vi "AR-Interlock-monitor.vi"() -> ()   [LabVIEW 2021]
uses:
  <vilib>/Instr/_visa.llb/VISA Flush IO Buffer Mask.ctl
panel:
  out "Output":string
  in  "Read":bool
  in  "stop":bool
  in  "Inlk Com":refnum<visa-resource-name>
  in  "error in":errorcluster
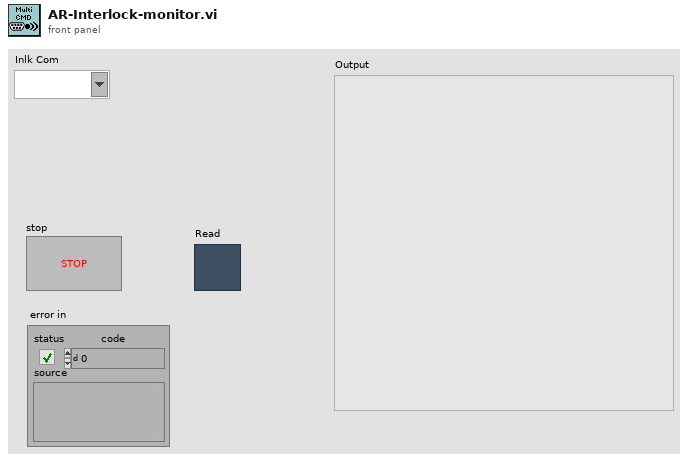
[diagram p1: front panel]
types:
  T1 = cluster{"Baud Rate":u32, "Parity":u16, "Data Bits":u16, "Serial Settings:Serial Flow Control":u16, "Serial Port":u16, "Serial Settings:Serial Stop Bits":u16}
  T2 = typedef "VISA Flush IO Buffer Mask.ctl" = u16
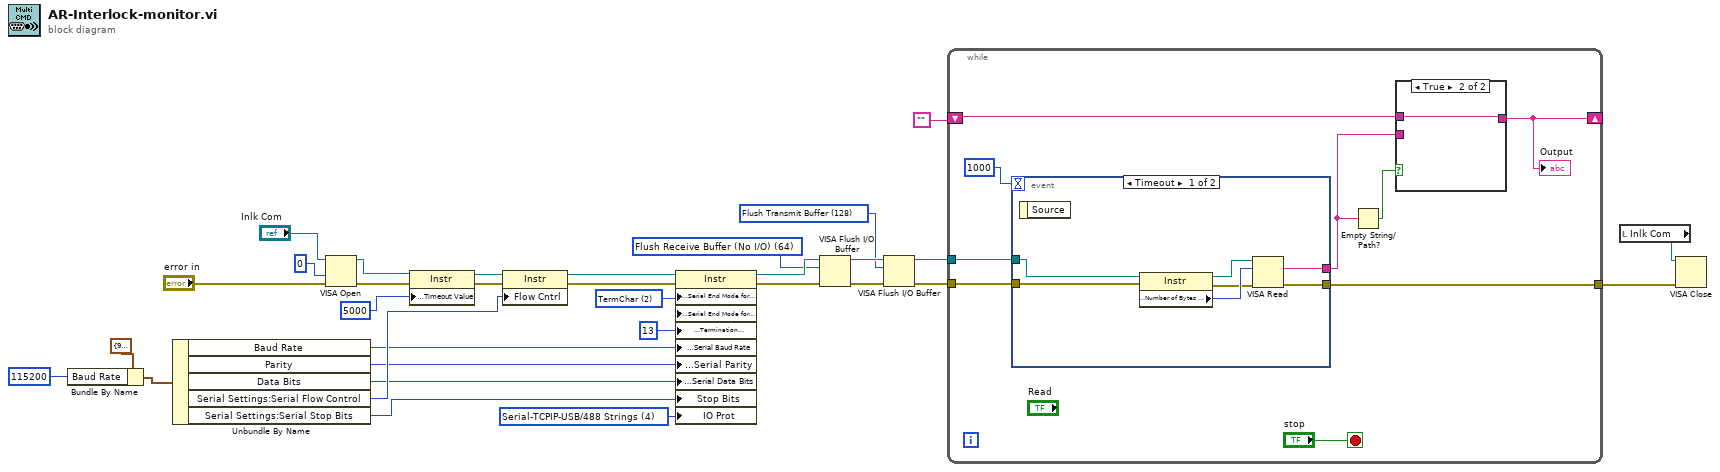
[diagram p0: block diagram]
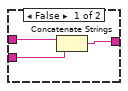
[diagram p2: hidden frame]
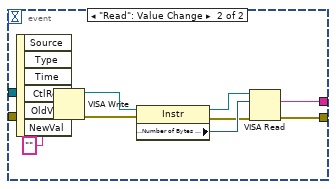
[diagram p3: hidden frame]
diagram:
  w7 = T2 128 items=["Flush Receive Buffer"=16, "Write Transmit Buffer to Device"=32, "Flush Receive Buffer (No I/O)"=64, "Flush Transmit Buffer"=128] ("Mask")
  w12 = T2 64 items=["Flush Receive Buffer"=16, "Write Transmit Buffer to Device"=32, "Flush Receive Buffer (No I/O)"=64, "Flush Transmit Buffer"=128] ("Mask")
  w23 = u16 2 items=["None", "LastBit", "TermChar"] ("Serial Settings:Serial End Mode for Reads")
  w19 = u16 4 items=["Normal"=1, "VXI/FDC"=2, "GPIB/HS488"=3, "Serial-TCPIP-USB/488 Strings"=4, "USBTMC/Vendor-Specific"=5] ("Message Based Settings:IO Protocol")
  n1 = Bundle By Name(cluster=T1 {"Baud Rate"=9600, "Parity"=0, "Data Bits"=8, "Serial Settings:Serial Flow Control"=0, "Serial Port"=6, "Serial Settings:Serial Stop Bits"=10} ("Serial Configuration"), "Baud Rate"=u32 115200) -> (w15:T1)
  n2 = Unbundle By Name(w15) -> ("Baud Rate"=w22:u32, "Parity"=w21:u16, "Data Bits"=w20:u16, "Serial Settings:Serial Flow Control"=w26:u16, "Serial Settings:Serial Stop Bits"=w18:u16)
  n3 = VISA Open(access mode=u32 0, error in (no error)="error in", VISA resource name="Inlk Com") -> (VISA resource name=w30:refnum<visa-resource-name>, error out=w31:errorcluster)  [unwired: 2 in]
  n4 = property on="Property Node" class="Instr"(reference=w30, error in=w31, "General Settings:Timeout Value"=u32 5000 ("Timeout [ms]")) -> (reference out=w28:refnum<visa-resource-name>, error out=w27:errorcluster)
  n5 = property on="Property Node" class="Instr"(reference=w28, error in=w27, "Flow Cntrl"=w26) -> (reference out=w25:refnum<visa-resource-name>, error out=w24:errorcluster)
  n6 = property on="Property Node" class="Instr"(reference=w25, error in=w24, "Serial Settings:Serial End Mode for Reads"=w23, "Serial Settings:Serial End Mode for Writes"=w23, "Message Based Settings:Termination Character"=u8 13, "Serial Settings:Serial Baud Rate"=w22, "Serial Settings:Serial Parity"=w21, "Serial Settings:Serial Data Bits"=w20, "Stop Bits"=w18, "IO Prot"=w19) -> (reference out=w14:refnum<visa-resource-name>, error out=w13:errorcluster)
  n7 = VISA Flush I/O Buffer(VISA resource name=w14, mask (16)=w12, error in (no error)=w13) -> (VISA resource name out=w11:refnum<visa-resource-name>, error out=w10:errorcluster)
  n8 = VISA Flush I/O Buffer(VISA resource name=w11, mask (16)=w7, error in (no error)=w10) -> (VISA resource name out=w8:refnum<visa-resource-name>, error out=w9:errorcluster)
  n9 = while {
    tunnel: w9 -> [w41]
    tunnel: w8 -> [w40]
    tunnel: [w37] -> w2
    shift-right: [w33] -> _
    shift-left: "" -> [w34]
    stop <- "stop" stop-if-true
    n10 = event shown="[0] Timeout" {
      selector: _ -> [_ _]
      dyn-events: _ -> [_ _]
      timeout: 1000 -> [_ _]
      tunnel: w41 -> [w49 w62]
      tunnel: w40 -> [w48 w61]
      tunnel: [w47 w55] -> w37
      tunnel: [w46 w54] -> w35
      event Timeout {
        n11 = event-data() -> ()  [unwired: 1 in, 1 out]
        n12 = property class="Instr"(reference=w48, error in=w49) -> (reference out=w52:refnum<visa-resource-name>, error out=w50:errorcluster, "Serial Settings:Number of Bytes at Serial Port"=w51:u32)
        n13 = VISA Read(VISA resource name=w52, byte count=w51, error in (no error)=w50) -> (read buffer=w46:string, error out=w47:errorcluster)  [unwired: 2 out]
      }
      event "Read": Value Change {
        n14 = event-data() -> ()  [unwired: 1 in, 6 out]
        n15 = VISA Write(VISA resource name=w61, write buffer="", error in (no error)=w62) -> (VISA resource name out=w60:refnum<visa-resource-name>, error out=w59:errorcluster)  [unwired: 1 out]
        n16 = property class="Instr"(reference=w60, error in=w59) -> (reference out=w58:refnum<visa-resource-name>, error out=w56:errorcluster, "Serial Settings:Number of Bytes at Serial Port"=w57:u32)
        n17 = VISA Read(VISA resource name=w58, byte count=w57, error in (no error)=w56) -> (read buffer=w54:string, error out=w55:errorcluster)  [unwired: 2 out]
      }
    }
    n18 = Empty String/Path?(string/path=w35) -> (empty?=w36:bool)
    n19 = case shown="True" w36 {
      tunnel: w35 -> [w44 _]
      tunnel: w34 -> [w43 w45]
      tunnel: [w42 w45] -> w33
      frame False {
        n20 = Concatenate Strings(w43, w44) -> (w42:string)
      }
      frame True {
      }
    }
    "Output" <- w33
  }
  n21 = local read "Inlk Com"() -> (w1:refnum<visa-resource-name>)
  n22 = VISA Close(VISA resource name=w1, error in (no error)=w2) -> ()  [unwired: 1 out]
